vi "enqueue_commands.vi"(8 "error in (no error)":errorcluster caption="错误输入（无错误）", 10 "command cluster":cluster{"cmd":T1, "cmd data":variant}, 11 "MotorSystem输入":refnum<class "MotorSystem.lvclass">) -> (0 "error out":errorcluster caption="错误输出", 3 "MotorSystem输出":refnum<class "MotorSystem.lvclass">)   [LabVIEW 2016, in "MotionControl_UFO_3DOF.lvlib" / "MotorSystem.lvclass"]
uses:
  <userlib>/MotionControl_UFO_3DOF/MotorSystem/MotorSystem.lvclass
  <userlib>/MotionControl_UFO_3DOF/MotorSystem/cmd_system.ctl
  <userlib>/MotionControl_UFO_3DOF/MotorSystem/MotorSystem.lvclass/MotorSystem.ctl
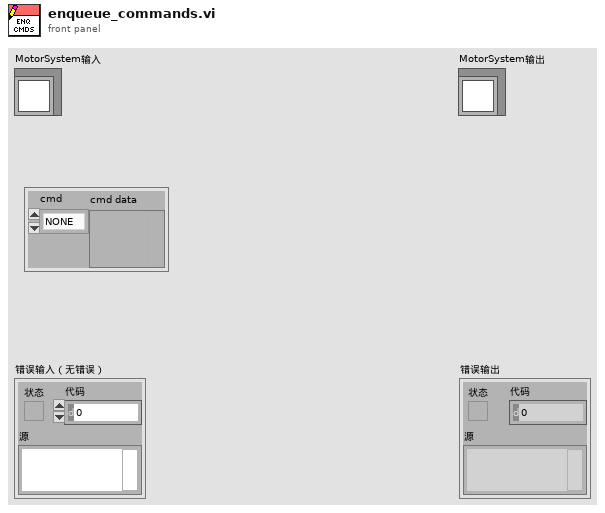
[diagram p1: front panel]
types:
  T1 = typedef "MotionControl_UFO_3DOF.lvlib/MotorSystem.lvclass/cmd_system.ctl" = enum16{"NONE", "MOVE_SYSTEM", "WAIT_UNTIL_MOVE_DONE", "EXIT", "WAIT_UNTIL_SELECTED_MOVE_DONE", "WAIT_A_TIME"}
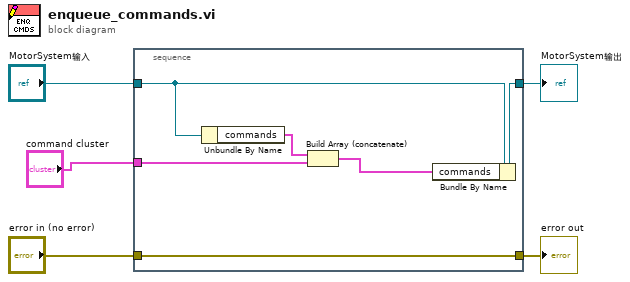
[diagram p0: block diagram]
diagram:
  n1 = stacked-sequence {
    tunnel: [w10] -> w5
    tunnel: [w11] -> w3
    tunnel: "MotorSystem输入" -> [w9]
    tunnel: "error in (no error)" -> [w10]
    tunnel: "command cluster" -> [w7]
    frame #0 {
      n2 = Unbundle By Name(w9) -> ("commands"=w8:cluster{"cmd":T1, "cmd data":variant}[])
      n3 = Build Array (concatenate)(w8, w7) -> (w6:cluster{"cmd":T1, "cmd data":variant}[])
      n4 = Bundle By Name(cluster=w9, "commands"=w6) -> (w11:refnum<class "MotorSystem.lvclass">)
    }
  }
  "error out" <- w5
  "MotorSystem输出" <- w3
